vi "SelectCprRutine.vi"(6 "CPR Number":string, 7 "error in":errorcluster, 8 "Journal Menu":refnum<vi>, 9 "Data Listbox":refnum<vi>, 10 "ProcessDataTreeMenu":refnum<vi>) -> (0 "error out":errorcluster)   [LabVIEW 2013, in "main.lvlib"]
uses:
  main.lvlib
  Globals/DataPathGlobalVariable.vi
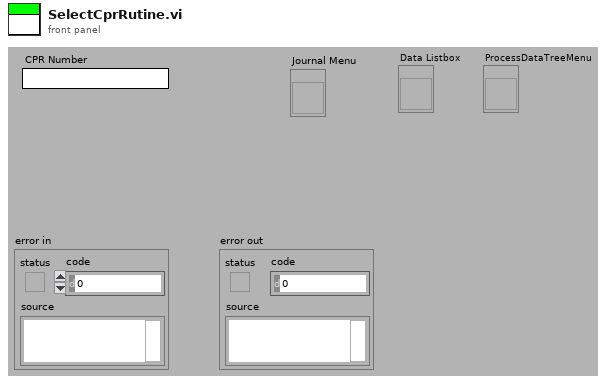
[diagram p1: front panel]
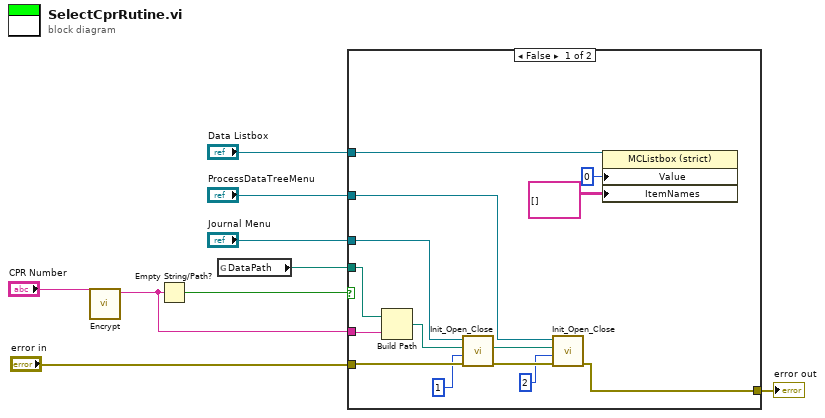
[diagram p0: block diagram]
diagram:
  n1 = call "Encrypt.vi"("Input"="CPR Number") -> ("Output"=w5:string)  [unwired: 10 in]
  n2 = Empty String/Path?(string/path=w5) -> (empty?=w9:bool)
  n3 = global read "DataPathGlobalVariable.vi" "DataPath"() -> (w4:path)
  n4 = case shown="False" w9 {
    tunnel: "error in" -> [w21 w23]
    tunnel: [w20 w23] -> w8
    tunnel: w5 -> [w19 _]
    tunnel: w4 -> [w15 _]
    tunnel: "Journal Menu" -> [w14 _]
    tunnel: "ProcessDataTreeMenu" -> [w13 _]
    tunnel: "Data Listbox" -> [w12 _]
    frame False {
      n5 = Build Path(base path=w15, name or relative path=w19) -> (appended path=w18:path)
      n6 = call "Init_Open_Close.vi"("error in"=w21, "Level"=1, "path to start the search"=w18, "Tree In"=w14) -> ("error out"=w22:errorcluster)  [unwired: 5 in, 2 out]
      n7 = call "Init_Open_Close.vi"("error in"=w22, "Level"=2, "path to start the search"=w18, "Tree In"=w13) -> ("error out"=w20:errorcluster)  [unwired: 5 in, 2 out]
      n8 = property class="MCListbox (strict)"(reference=w12, "Value"=0, "ItemNames"=string[][] [] ("Item Names")) -> ()  [unwired: 1 in, 2 out]
    }
    frame True {
    }
  }
  "error out" <- w8
